vi "ProcessData.vi"(8 "error in (no error)":errorcluster, 9 "State":T1, 10 "Analog Data":T3, 11 "DotMappingExperiment in":refnum<class "DotMappingExperiment.lvclass">) -> (0 "error out":errorcluster, 1 "Fixated":bool, 2 "Trigger":T2=enum."Broke Fixation", 3 "DotMappingExperiment out":refnum<class "DotMappingExperiment.lvclass">)   [LabVIEW 2010, in "DotMappingExperiment.lvclass"]
uses:
  DotMappingExperiment.lvclass
  Core SubVIs/Controls/TYPE - Analog Data.ctl
  Trial Based Experiment Statechart/Trial Based Experiment.lvsc/Trigger.ctl
  Trial Based Experiment Statechart/Trial Based Experiment.lvsc/State.ctl
  <vilib>/measure/madcrms.llb/Basic Averaged DC-RMS for 1 Chan.vi
  Core SubVIs/Core SubVIs.lvlib
  <vilib>/measure/NI_MAPro.lvlib
  Trial Based Experiment Statechart/Trial Based Experiment.lvsc
panel:
  in  "Adjustment Rate":dbl=0.02
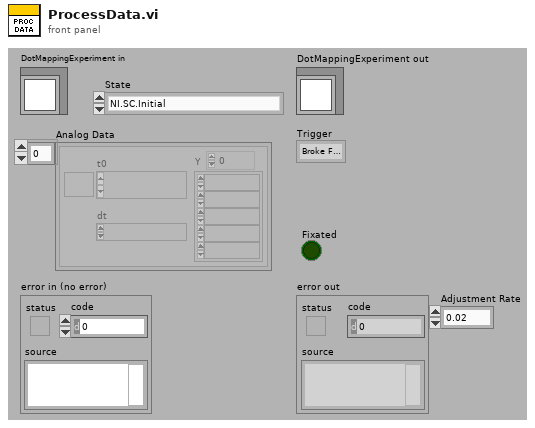
[diagram p1: front panel]
types:
  T1 = typedef "Trial Based Experiment.lvsc/State.ctl" = enum16{"NI.SC.Initial", "NI.SC.History", "NI.SC.ShallowHistory", "NI.SC.Terminal", "Cleanup", "State", "State\\Region\\Pause", "State\\Region\\Response Period", "State\\Region\\Delay Period", "State\\Region\\Hold Fixation", "State\\Region\\Acquire Fixation", "State\\Region\\Abort Trial", "State\\Region\\End Trial", "State\\Region\\Intertrial", "State\\Region\\Start Trial"}
  T2 = typedef "Trial Based Experiment.lvsc/Trigger.ctl" = enum16{"NULL", "Fixated", "Broke Fixation", "Stop", "Correct Response", "Incorrect Response", "Timeout"}
  T3 = typedef "Core SubVIs.lvlib/TYPE - Analog Data.ctl" = waveform(dbl)[]
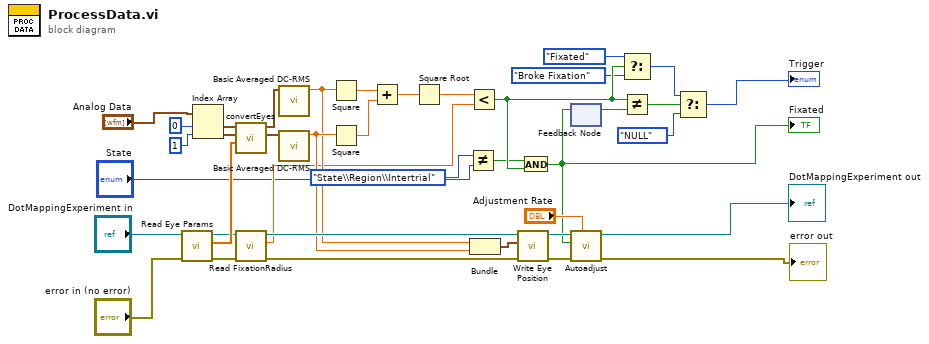
[diagram p0: block diagram]
diagram:
  n1 = call-dynamic "Read Eye Params.vi"("error in (no error)"="error in (no error)", "TrialBasedExperiment in"="DotMappingExperiment in") -> ("error out"=w28:errorcluster, "Eye Params"=w17:dbl[], "TrialBasedExperiment out"=w6:refnum<class "DotMappingExperiment.lvclass">)  [unwired: 7 in]
  n2 = Index Array(array="Analog Data", index #1=0 ("index"), index #2=1 ("index")) -> (element #1=w10:waveform(dbl), element #2=w9:waveform(dbl))
  n3 = call "convertEyes.vi"("Params"=w17, "Vertical"=w9, "Horizontal"=w10) -> ("Vertical Calibrated"=w14:waveform(dbl), "Horizontal Calibrated"=w15:waveform(dbl))  [unwired: 7 in]
  n4 = call-dynamic "Read FixationRadius.vi"("error in (no error)"=w28, "MatlabExperiment in"=w6) -> ("error out"=w35:errorcluster, "FixationRadius"=w27:dbl, "MatlabExperiment out"=w32:refnum<class "DotMappingExperiment.lvclass">)  [unwired: 7 in]
  n5 = call-poly <vilib>:"Basic Averaged DC-RMS.vi"("signal in"=w15) -> ("DC value"=w29:dbl)  [unwired: 7 in, 3 out]
  n6 = call-poly <vilib>:"Basic Averaged DC-RMS.vi"("signal in"=w14) -> ("DC value"=w30:dbl)  [unwired: 7 in, 3 out]
  n7 = Square(x=w29) -> (x^2=w21:dbl)
  n8 = Square(x=w30) -> (x^2=w22:dbl)
  n9 = Add(x=w21, y=w22) -> (x+y=w23:dbl)
  n10 = Square Root(x=w23) -> (sqrt(x)=w24:dbl)
  n11 = Not Equal?(x=State."State\\Region\\Intertrial", y="State") -> (x != y?=w38:bool)
  n12 = Less?(x=w24, y=w27) -> (x < y?=w39:bool)
  n13 = Bundle("DC value"=w29, "DC value"=w30) -> (w31:cluster{"DC value":dbl, "DC value":dbl})  [unwired: 1 in]
  n14 = call-dynamic "Write Eye Position.vi"("error in (no error)"=w35, "Eye Position"=w31, "TrialBasedExperiment in"=w32) -> ("error out"=w36:errorcluster, "TrialBasedExperiment out"=w33:refnum<class "DotMappingExperiment.lvclass">)  [unwired: 7 in]
  n15 = And(x=w38, y=w39) -> (x .and. y?=w3:bool)
  "Fixated" <- w3
  n16 = feedback #1() -> (w20:bool)  [unwired: 1 in]
  n17 = feedback-in #1(w3) -> ()
  n18 = call-dynamic "Autoadjust.vi"("Adjustment Rate"="Adjustment Rate", "error in (no error)"=w36, "Fixated"=w3, "TrialBasedExperiment in"=w33) -> ("error out"=→"error out":errorcluster, "TrialBasedExperiment out"=→"DotMappingExperiment out":refnum<class "DotMappingExperiment.lvclass">)  [unwired: 6 in]
  n19 = Select(t=Trigger."Fixated" ("Trigger"), s=w39, f=Trigger."Broke Fixation" ("Trigger")) -> (s? t:f=w19:T2)
  n20 = Not Equal?(x=w39, y=w20) -> (x != y?=w26:bool)
  n21 = Select(t=w19, s=w26, f=Trigger."NULL" ("Trigger")) -> (s? t:f=→"Trigger":T2)
